vi "set valves from status.vi"(0 "system status in":T1={"system state"=enum."Empty & Closed", "fuel level"=0.0, "LOX level"=0.0, "system warnings"={"oxidizer overpress"=FALSE, "oxidizer leak"=FALSE, "fuel overpress"=FALSE, "fuel leak"=FALSE}, "valves"={"fuel load"=FALSE, "fuel return"=FALSE, "fuel comb"=FALSE, "fuel dump"=FALSE, "LOX load"=FALSE, "LOX return"=FALSE, "LOX comb"=FALSE, "LOX dump"=FALSE}, "ignition"=FALSE}) -> (12 "fuel load":u16, 13 "LOX dump":u16, 14 "fuel return":u16, 15 "fuel comb":u16, 16 "fuel dump":u16, 17 "LOX load":u16, 18 "LOX return":u16, 19 "LOX comb":u16)   [LabVIEW 2017]
doc: "This subVI reads the desired valve states in the system status cluster and outputs the integer values to each individual valve. It is used for updating the front panel.\n\nPaul K Dixon\nP350\nCSUSB"
uses:
  typedefs/sysyem status.ctl
  typedefs/system state.ctl
  typedefs/rocket system warnings.ctl
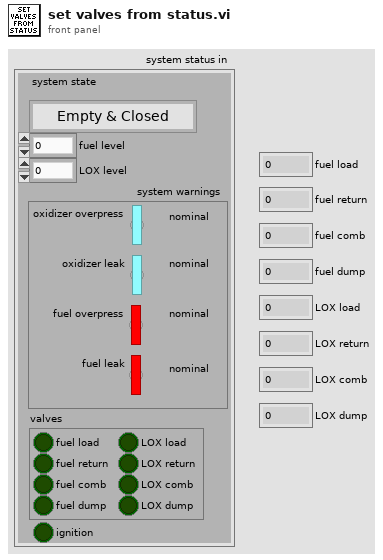
[diagram p1: front panel]
types:
  T1 = typedef "sysyem status.ctl" = cluster{"system state":T2, "fuel level":dbl, "LOX level":dbl, "system warnings":T3, "valves":cluster{"fuel load":bool, "fuel return":bool, "fuel comb":bool, "fuel dump":bool, "LOX load":bool, "LOX return":bool, "LOX comb":bool, "LOX dump":bool}, "ignition":bool}
  T2 = typedef "system state.ctl" = enum16{"Hold", "Empty & Closed", "Launch", "Return Fuel", "Return LOX", "Loading Lox", "Loading Fuel", "Shutdown", "Abort"}
  T3 = typedef "rocket system warnings.ctl" = cluster{"oxidizer overpress":bool, "oxidizer leak":bool, "fuel overpress":bool, "fuel leak":bool}
  T4 = cluster{"fuel load":bool, "fuel return":bool, "fuel comb":bool, "fuel dump":bool, "LOX load":bool, "LOX return":bool, "LOX comb":bool, "LOX dump":bool}
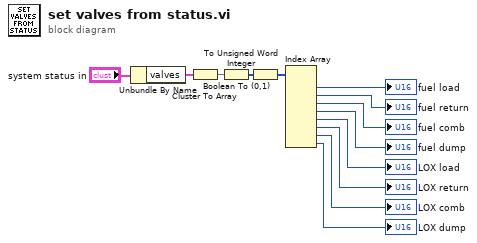
[diagram p0: block diagram]
diagram:
  n1 = Unbundle By Name("system status in") -> ("valves"=w12:T4)
  n2 = Cluster To Array(cluster=w12) -> (array=w11:bool[])
  n3 = Boolean To (0,1)(Boolean=w11) -> (0, 1=w10:i16[])
  n4 = To Unsigned Word Integer(number=w10) -> (unsigned 16bit integer=w9:u16[])
  n5 = Index Array(array=w9) -> (element #1=→"fuel load":u16, element #2=→"fuel return":u16, element #3=→"fuel comb":u16, element #4=→"fuel dump":u16, element #5=→"LOX load":u16, element #6=→"LOX return":u16, element #7=→"LOX comb":u16, element #8=→"LOX dump":u16)  [unwired: 8 in]
